vi "TCP Open.vi"   [LabVIEW 2013, in "TCP.lvclass"]
uses:
  TCP.lvclass
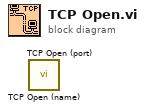
[diagram p0: block diagram]
diagram:
  n1 = call "TCP Open (name).vi"() -> ()  [unwired: 10 in, 2 out]
  n2 = call "TCP Open (port).vi"() -> ()  [unwired: 10 in, 2 out]
